vi "Create Instrument.vi"(8 "error in":errorcluster, 11 "Instrument Factory in":refnum<class "Instrument Factory.lvclass">) -> (0 "error out":errorcluster, 3 "Instrument Factory out":refnum<class "Instrument Factory.lvclass">)   [LabVIEW 2025]
uses:
  Instrument Factory.lvclass
  Instrument Factory.lvclass/Instrument Factory.ctl
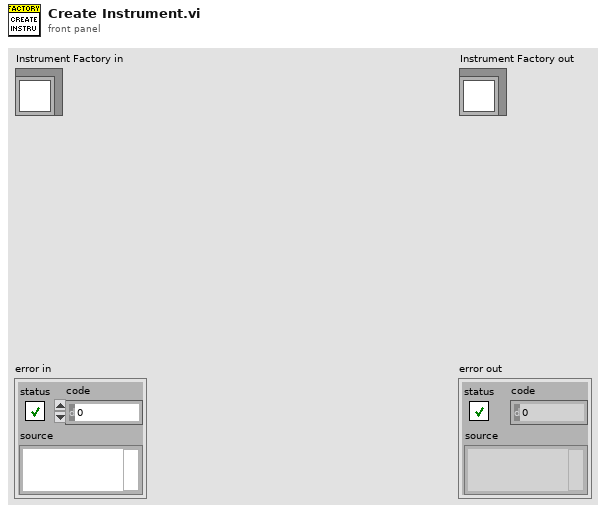
[diagram p1: front panel]
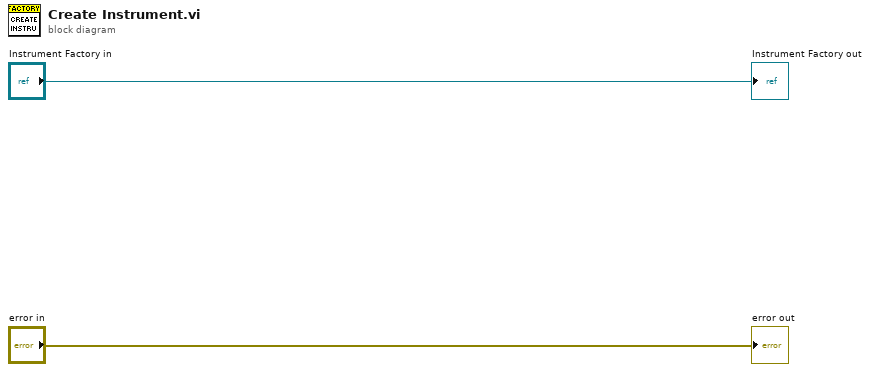
[diagram p0: block diagram]
diagram:
  "error out" <- "error in"
  "Instrument Factory out" <- "Instrument Factory in"
